vi "Has Disconnected.vi"(8 "error in (no error)":errorcluster, 11 "Low Level Connection in":refnum<class "Low Level Connection.lvclass">) -> (0 "error out":errorcluster, 2 "has disconnected?":bool, 3 "Low Level Connection out":refnum<class "Low Level Connection.lvclass">)   [LabVIEW 2020, in "NI_SFTP.lvlib" / "Low Level Connection.lvclass"]
uses:
  <vilib>/net/SFTP/Low Level Connection/Low Level Connection.lvclass
  <vilib>/net/SFTP/Low Level Connection/Low Level Connection.lvclass/Low Level Connection.ctl
  <vilib>/Subprocess/Buffered Subprocess/Buffered Subprocess.lvclass
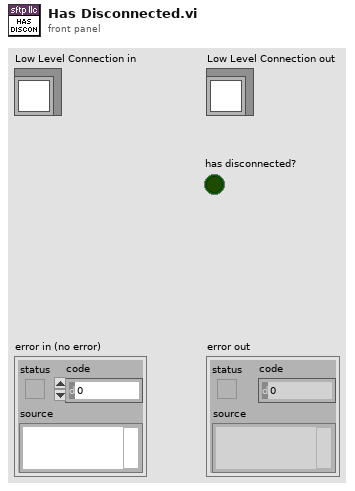
[diagram p1: front panel]
types:
  T1 = cluster{"subprocess":refnum<class "Buffered Subprocess.lvclass">, "read stdout":refnum<class "Bytestream.lvclass">}
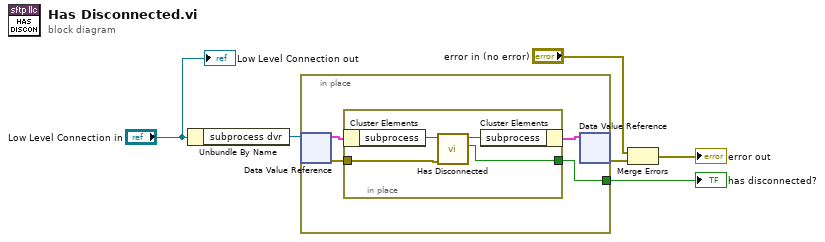
[diagram p0: block diagram]
diagram:
  n1 = Unbundle By Name("Low Level Connection in") -> ("subprocess dvr"=w2:refnum<data-value>)
  n2 = in-place {
    in-place-border: [w7] -> w3
    n3 = in-place-dvr #1(w2) -> (w10:T1, w9:errorcluster)
    n4 = in-place {
      in-place-border: w9 -> [w13]
      in-place-border: [w11] -> w7
      n5 = in-place-cluster #2(w10) -> ("subprocess"=w14:refnum<class "Buffered Subprocess.lvclass">)
      n6 = call <vilib>:"Has Disconnected.vi"("error in (no error)"=w13, "Buffered Subprocess in"=w14) -> ("disconnected?"=w11:bool, "Buffered Subprocess out"=w12:refnum<class "Buffered Subprocess.lvclass">)  [unwired: 7 in, 1 out]
      n7 = in-place-cluster #2("subprocess"=w12) -> (w8:T1)
    }
    n8 = in-place-dvr #1(w8) -> (w1:errorcluster)  [unwired: 1 out]
  }
  "has disconnected?" <- w3
  n9 = Merge Errors("error in (no error)", w1) -> (→"error out":errorcluster)
  "Low Level Connection out" <- "Low Level Connection in"
